vi "实验2_3.vi"() -> ()   [LabVIEW 2018]
panel:
  out "one":dbl[](array[numeric])
  out "min":dbl
  out "max":dbl
  out "size":dbl[](array[numeric])
  out "T":dbl[][](array[numeric])
  out "init":dbl[][](array[numeric])
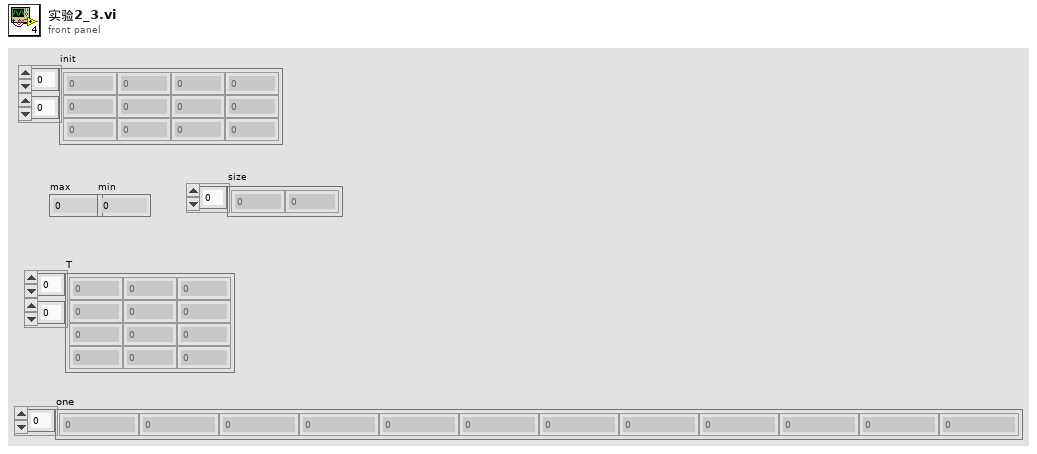
[diagram p1: front panel]
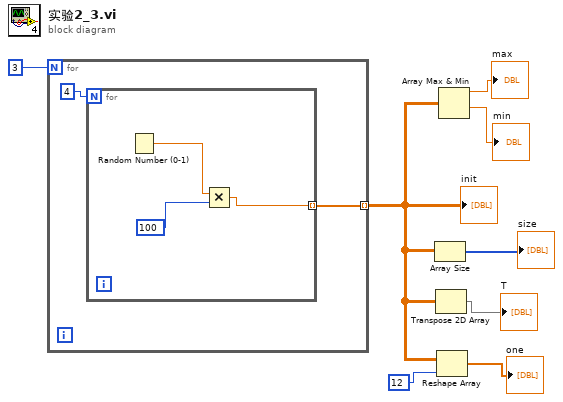
[diagram p0: block diagram]
diagram:
  n1 = for {
    N: 3 -> [_]
    tunnel: [w10] -> w3 mode=indexing
    n2 = for {
      N: 4 -> [_]
      tunnel: [w11] -> w10 mode=indexing
      n3 = Random Number (0-1)() -> (number: 0 to 1=w13:dbl)
      n4 = Multiply(x=w13, y=100) -> (x*y=w11:dbl)
    }
  }
  "init" <- w3
  n5 = Array Size(array=w3) -> (size(s)=→"size":i32[])
  n6 = Transpose 2D Array(2D array=w3) -> (transposed array=→"T":dbl[][])
  n7 = Reshape Array(w3, 12) -> (→"one":dbl[])
  n8 = Array Max & Min(array=w3) -> (max value=→"max":dbl, min value=→"min":dbl)  [unwired: 2 out]
